vi "OW Init.vi"(7 "EnInternalPull":u8, 9 "ResetTimeUs":u32, 10 "ChannelMask":u32, 11 "DevHandle":i32) -> (3 "function return":i32)   [LabVIEW 2010, in "usb2ow.lvlib"]
doc: "int WINAPI OW_Init(int DevHandle, unsigned int ChannelMask, unsigned int ResetTimeUs,unsigned char EnInternalPull);"
uses:
  usb2ow.lvlib
  USB2XXX/trunk/USB2XXX/USB2XXX/vs2010/Release/USB2XXX.dll
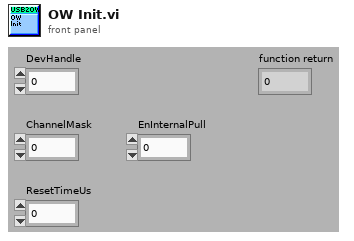
[diagram p1: front panel]
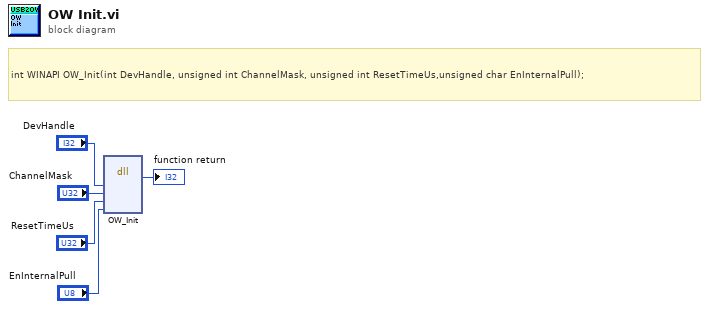
[diagram p0: block diagram]
diagram:
  # "int WINAPI OW_Init(int DevHandle, unsigned int ChannelMask, unsigned int ResetTimeUs,unsigned char EnInternalPull);"
  n1 = dll-call lib="E:/OtherWork/STM32/USB2XXX/trunk/USB2XXX/USB2XXX/vs2010/Release/USB2XXX.*" fn="OW_Init"("DevHandle"="DevHandle", "ChannelMask"="ChannelMask", "ResetTimeUs"="ResetTimeUs", "EnInternalPull"="EnInternalPull") -> (→"function return":i32)  [unwired: 7 in, 2 out]
